vi "SortPriority.vi"(8 "error in (no error)":errorcluster, 11 "Array in":T1[](array[typedef])) -> (0 "error out":errorcluster, 3 "Array out":T1[](array[typedef]))   [LabVIEW 2017, in "Client.lvlib" / "ParserSorter.lvlib"]
doc: "Check If Days Open > 0,1 and calculate Score based on Prio specific Base Values"
uses:
  ParserSorter.lvlib
  SR Data.ctl
  AE Group.ctl
  SR Status.ctl
  SR Level.ctl
  SR Type.ctl
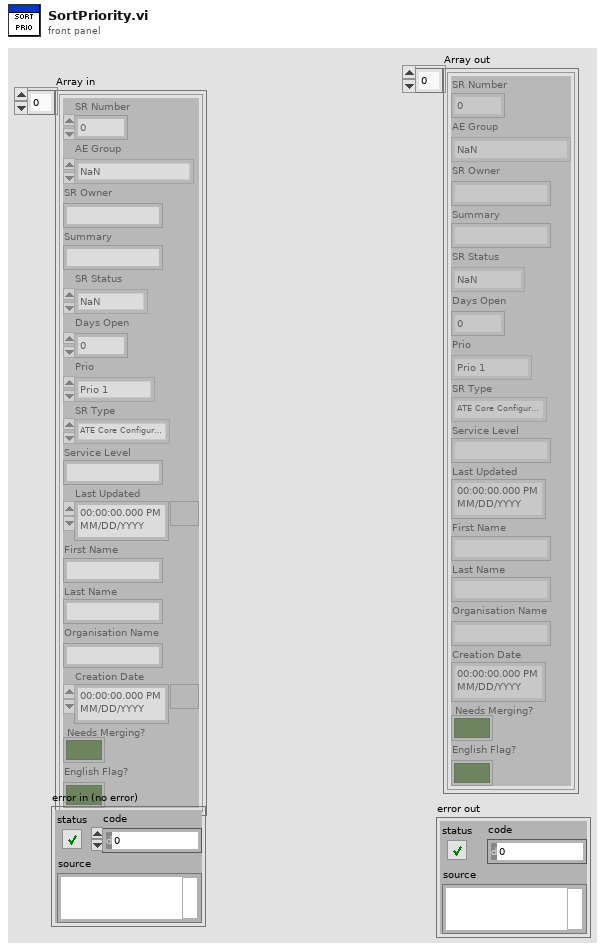
[diagram p1: front panel]
types:
  T1 = typedef "Client.lvlib/ParserSorter.lvlib/SR Data.ctl" = cluster{"SR Number":i64, "AE Group":T2, "SR Owner":string, "Summary":string, "SR Status":T3, "Days Open":dbl, "Prio":T4, "SR Type":T5, "Service Level":string, "Last Updated":timestamp, "First Name":string, "Last Name":string, "Organisation Name":string, "Creation Date":timestamp, "Needs Merging?":bool, "English Flag?":bool}
  T2 = typedef "Client.lvlib/ParserSorter.lvlib/AE Group.ctl" = enum32{"NaN", "AE-Germany", "AE-Poland", "AE-Switzerland", "AE-Czech Republic", "AE-Hungary", "AE-Romania", "AE-Slovakia", "AE-Slovenia"}
  T3 = typedef "Client.lvlib/ParserSorter.lvlib/SR Status.ctl" = enum32{"NaN", "Caller Abandoned", "Created in Error", "Declined to Purchase Support", "Expired", "Forum Resolved AE", "Forum Resolved Customer", "IN WORK", "IN WORK Collab with AES", "IN WORK Collab with PSE", "IN WORK Collab with SE", "IN WORK Escalation", "IN WORK Customer Added Note", "Open", "Potentially Resolved", "POC Resolved", "Resolved", "RMA Waiting on Customer", "RMA Open", "RMA In Progress", "RMA Closed - DOA", "RMA Closed", "RMA Approved for Return", "Project Complete", "Presumed Resolved", "IN WORK Wait on Customer"}
  T4 = typedef "Client.lvlib/ParserSorter.lvlib/SR Level.ctl" = enum16{"Prio 1", "Prio 2", "Prio 3", "Prio 4"}
  T5 = typedef "Client.lvlib/ParserSorter.lvlib/SR Type.ctl" = enum32{"NaN", "ATE Core Configurations (BYOATE)", "Activation", "BioBench", "CAN", "CM C Series", "Calibration", "Consulting Services", "CounterTimer", "DAQExpress", "DASYLab", "DIAdem", "DMM", "DSA HW", "Digital_IO", "FIRST (NIC Only)", "FieldBus", "FieldPoint", "Functional Savety", "GATI", "GPIB", "HMI and Industrial PCs", "HiQ", "HighSpeedDigital_IO", "IMAQ", "IOTech Vibration", "Industrial Communications", "InsightCM", "LV", "LV CD&Sim", "LV Comms", "LV Controls Add-Ons", "LV Embedded", "LV MathScript RT", "LV NXG", "LV NXT", "LVDSC", "LVFPGA", "LVPDA and LV Touch Panel", "LVRT", "LabWindows_CVI", "Lookout", "MATRIXx", "MStudioDotNet", "MStudioVisualBasic", "MStudioVisualC", "Measure (Legacy)", "Motion", "MultifunctionDAQ", "Multimedia Test HW/SW", "Multisim (EWB)", "NI Update Service", "OPC Servers", "Optical (OSI)", "PXI Controllers, Chassis, MXI", "PXI Timing and Sync", "Power Supplies and SMUs", "Powertrain Controls", "RAID", "RF", "RF Software", "RIO", "SC Express", "SCC", "SCXI", "SPEEDY-33 (Hyperception)", "STS", "ScopeDigitizers", "Serial", "Signal Sources", "SignalCondOther", "SignalExpress", "Software Defined Intruments", "Sound and Vibration SW", "Switch Executive", "Switches", "TestStand", "USRP", "Ultiboard (EWB)", "VBench", "VI Logger", "VXI_MXI", "VeriStand", "VisionSW", "VolumeLicenseMgr", "WSN", "Web UI Builder", "myRIO"}
  T6 = cluster{"Prio 1":cluster{"Days Open":dbl, "SR Number":i64}[], "Prio 2":cluster{"Days Open":dbl, "SR Number":i64}[], "Prio 3":cluster{"Days Open":dbl, "SR Number":i64}[], "Prio 4":cluster{"Days Open":dbl, "SR Number":i64}[]}
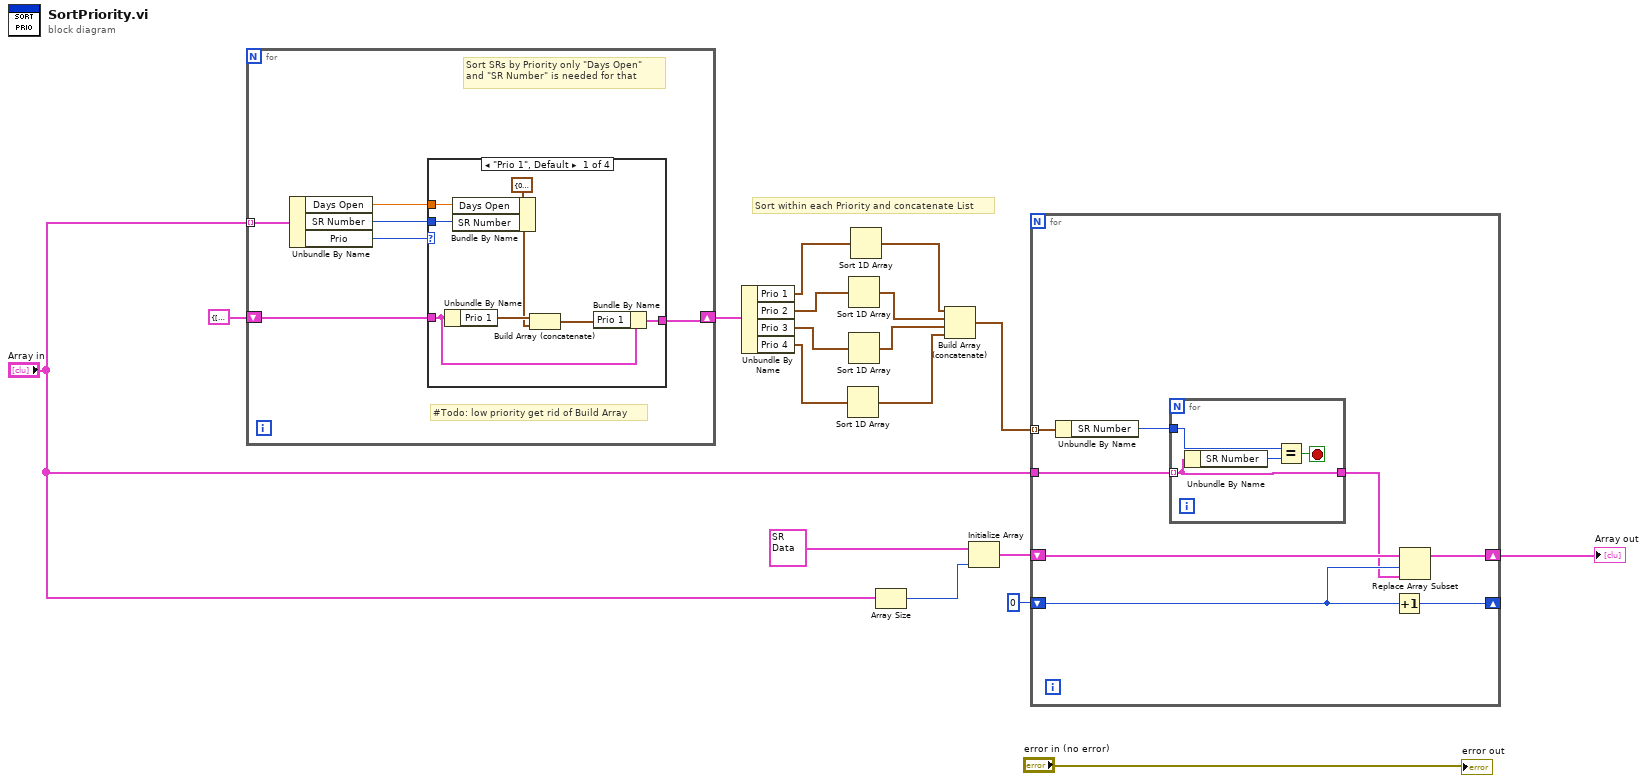
[diagram p0: block diagram]
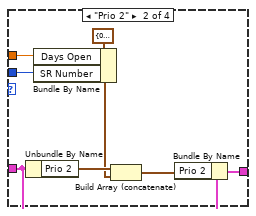
[diagram p2: hidden frame]
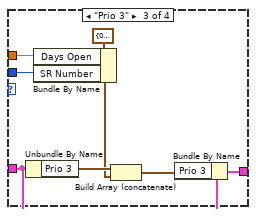
[diagram p3: hidden frame]
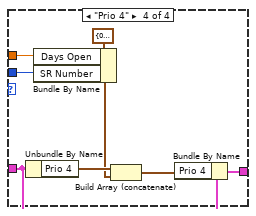
[diagram p4: hidden frame]
diagram:
  # "Sort within each Priority and concatenate List"
  n1 = for {
    tunnel: "Array in" -> [w22] mode=indexing
    shift-right: [w21] -> w17
    shift-left: T6 {"Prio 1"=[], "Prio 2"=[], "Prio 3"=[], "Prio 4"=[]} -> [w23]
    # "Sort SRs by Priority only \"Days Open\" \nand \"SR Number\" is needed for that"
    # "#Todo: low priority get rid of Build Array"
    n2 = Unbundle By Name(w22) -> ("Days Open"=w20:dbl, "SR Number"=w19:i64, "Prio"=w24:T4)
    n3 = case shown="\"Prio 1\", Default" w24 {
      tunnel: w23 -> [w31 w39 w47 w55]
      tunnel: [w29 w37 w45 w53] -> w21
      tunnel: w20 -> [w27 w35 w43 w51]
      tunnel: w19 -> [w26 w34 w42 w50]
      frame "Prio 1", Default {
        n4 = Unbundle By Name(w31) -> ("Prio 1"=w32:cluster{"Days Open":dbl, "SR Number":i64}[])
        n5 = Bundle By Name(cluster=cluster{"Days Open":dbl, "SR Number":i64} {"Days Open"=0.0, "SR Number"=0}, "Days Open"=w27, "SR Number"=w26) -> (w25:cluster{"Days Open":dbl, "SR Number":i64})
        n6 = Build Array (concatenate)(w32, w25) -> (w30:cluster{"Days Open":dbl, "SR Number":i64}[])
        n7 = Bundle By Name(cluster=w31, "Prio 1"=w30) -> (w29:T6)
      }
      frame "Prio 2" {
        n8 = Unbundle By Name(w39) -> ("Prio 2"=w40:cluster{"Days Open":dbl, "SR Number":i64}[])
        n9 = Bundle By Name(cluster=cluster{"Days Open":dbl, "SR Number":i64} {"Days Open"=0.0, "SR Number"=0}, "Days Open"=w35, "SR Number"=w34) -> (w33:cluster{"Days Open":dbl, "SR Number":i64})
        n10 = Build Array (concatenate)(w40, w33) -> (w38:cluster{"Days Open":dbl, "SR Number":i64}[])
        n11 = Bundle By Name(cluster=w39, "Prio 2"=w38) -> (w37:T6)
      }
      frame "Prio 3" {
        n12 = Unbundle By Name(w47) -> ("Prio 3"=w48:cluster{"Days Open":dbl, "SR Number":i64}[])
        n13 = Bundle By Name(cluster=cluster{"Days Open":dbl, "SR Number":i64} {"Days Open"=0.0, "SR Number"=0}, "Days Open"=w43, "SR Number"=w42) -> (w41:cluster{"Days Open":dbl, "SR Number":i64})
        n14 = Build Array (concatenate)(w48, w41) -> (w46:cluster{"Days Open":dbl, "SR Number":i64}[])
        n15 = Bundle By Name(cluster=w47, "Prio 3"=w46) -> (w45:T6)
      }
      frame "Prio 4" {
        n16 = Unbundle By Name(w55) -> ("Prio 4"=w56:cluster{"Days Open":dbl, "SR Number":i64}[])
        n17 = Bundle By Name(cluster=cluster{"Days Open":dbl, "SR Number":i64} {"Days Open"=0.0, "SR Number"=0}, "Days Open"=w51, "SR Number"=w50) -> (w49:cluster{"Days Open":dbl, "SR Number":i64})
        n18 = Build Array (concatenate)(w56, w49) -> (w54:cluster{"Days Open":dbl, "SR Number":i64}[])
        n19 = Bundle By Name(cluster=w55, "Prio 4"=w54) -> (w53:T6)
      }
    }
  }
  n20 = Unbundle By Name(w17) -> ("Prio 1"=w16:cluster{"Days Open":dbl, "SR Number":i64}[], "Prio 2"=w15:cluster{"Days Open":dbl, "SR Number":i64}[], "Prio 3"=w14:cluster{"Days Open":dbl, "SR Number":i64}[], "Prio 4"=w13:cluster{"Days Open":dbl, "SR Number":i64}[])
  n21 = Sort 1D Array(array=w13) -> (sorted array=w9:cluster{"Days Open":dbl, "SR Number":i64}[])
  n22 = Sort 1D Array(array=w15) -> (sorted array=w11:cluster{"Days Open":dbl, "SR Number":i64}[])
  n23 = Sort 1D Array(array=w14) -> (sorted array=w10:cluster{"Days Open":dbl, "SR Number":i64}[])
  n24 = Sort 1D Array(array=w16) -> (sorted array=w12:cluster{"Days Open":dbl, "SR Number":i64}[])
  n25 = Array Size(array="Array in") -> (size(s)=w6:i32)
  n26 = Build Array (concatenate)(w12, w11, w10, w9) -> (w8:cluster{"Days Open":dbl, "SR Number":i64}[])
  n27 = Initialize Array(T1 {"SR Number"=0, "AE Group"=enum."NaN", "SR Owner"="", "Summary"="", "SR Status"=enum."NaN", "Days Open"=0.0, "Prio"=enum."Prio 1", "SR Type"=enum."ATE Core Configurations (BYOATE)", "Service Level"="", "Last Updated"=timestamp(0 s since 1904-01-01), "First Name"="", "Last Name"="", "Organisation Name"="", "Creation Date"=timestamp(0 s since 1904-01-01), "Needs Merging?"=FALSE, "English Flag?"=FALSE} ("SR Number"), w6) -> (w5:T1[])
  n28 = for {
    shift-right: [w60] -> w2
    shift-left: w5 -> [w61]
    tunnel: w8 -> [w63] mode=indexing
    shift-right: [w58] -> _
    shift-left: 0 ("size(s)") -> [w59]
    tunnel: "Array in" -> [w64]
    n29 = Unbundle By Name(w63) -> ("SR Number"=w62:i64)
    n30 = for {
      tunnel: w64 -> [w65] mode=indexing
      tunnel: w62 -> [w68]
      tunnel: [w65] -> w57
      stop <- w66 stop-if-true
      n31 = Unbundle By Name(w65) -> ("SR Number"=w67:i64)
      n32 = Equal?(x=w68, y=w67) -> (x = y?=w66:bool)
    }
    n33 = Increment(x=w59) -> (x+1=w58:i32)
    n34 = Replace Array Subset(array=w61, new element=w57, index=w59) -> (w60:T1[])
  }
  "Array out" <- w2
  "error out" <- "error in (no error)"
